vi "GamePlayfield_DetectCollision.vi"(1 "Origin":i16, 4 "Tetromino":u8, 8 "AdditionalChecks":cluster{"LeftBorder":bool, "RightBorder":bool}, 9 "Player":u8) -> (16 "Collision":bool)   [LabVIEW 2018]
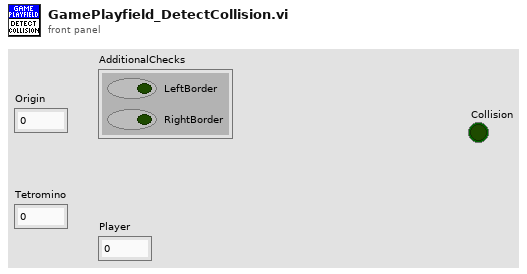
[diagram p1: front panel]
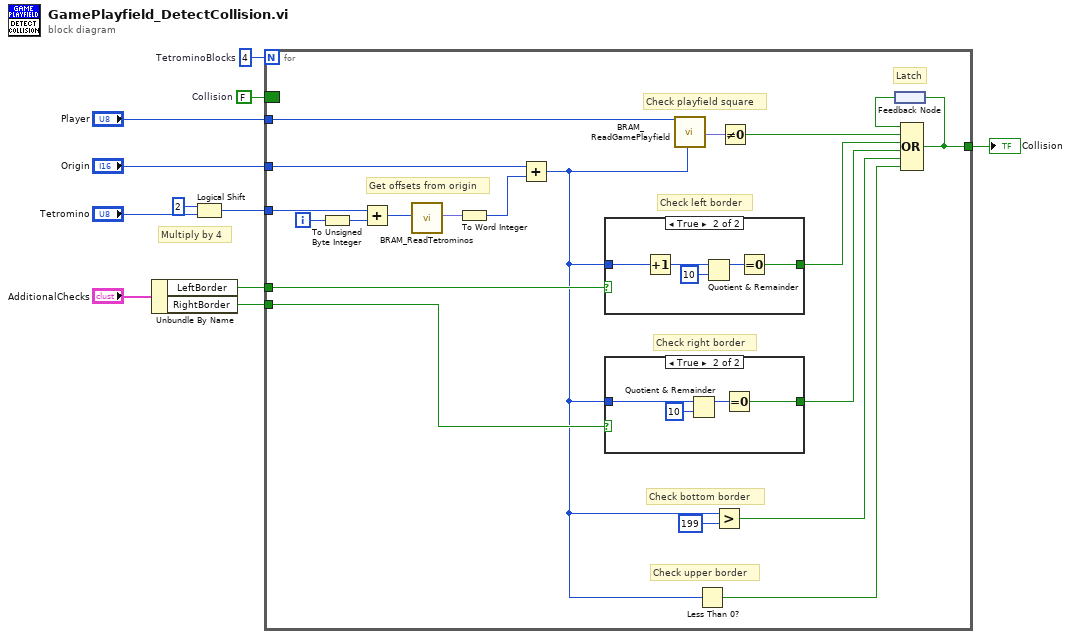
[diagram p0: block diagram]
diagram:
  w5 = FALSE  # Collision
  w9 = 4  # TetrominoBlocks
  # "Multiply by 4"
  n1 = Unbundle By Name("AdditionalChecks") -> ("LeftBorder"=w2:bool, "RightBorder"=w1:bool)
  n2 = Logical Shift(y=i16 2, x="Tetromino") -> (x << y=w8:u8)
  n3 = for {
    N: w9 -> [_]
    tunnel: w8 -> [w30]
    tunnel: "Origin" -> [w27]
    tunnel: [w24] -> w6
    border: w5 -> [_]
    tunnel: "Player" -> [w31]
    tunnel: w2 -> [w17]
    tunnel: w1 -> [w16]
    i -> [w29]
    # "Check upper border"
    # "Get offsets from origin"
    # "Check bottom border"
    # "Check right border"
    # "Check left border"
    # "Check playfield square"
    # "Latch"
    n4 = To Unsigned Byte Integer(number=w29) -> (unsigned 8bit integer=w28:u8)
    n5 = Add(x=w30, y=w28) -> (x+y=w21:u8)
    n6 = call "BRAM_ReadTetrominos.vi"("Address"=w21) -> ("Data"=w26:fxp<+,6,6>)  [unwired: 18 in]
    n7 = To Word Integer(number=w26) -> (16bit integer=w22:i16)
    n8 = Add(x=w27, y=w22) -> (x+y=w13:i16)
    n9 = case shown="True" w17 {
      tunnel: [_ w38] -> w23
      tunnel: w13 -> [_ w36]
      frame False {
      }
      frame True {
        n10 = Increment(x=w36) -> (x+1=w37:i16)
        n11 = Quotient & Remainder(x=w37, y=i16 10) -> (x-y*floor(x/y)=w40:i16)  [unwired: 1 out]
        n12 = Equal To 0?(x=w40) -> (x = 0?=w38:bool)
      }
    }
    n13 = case shown="True" w16 {
      tunnel: [_ w33] -> w18
      tunnel: w13 -> [_ w32]
      frame False {
      }
      frame True {
        n14 = Quotient & Remainder(x=w32, y=i16 10) -> (x-y*floor(x/y)=w35:i16)  [unwired: 1 out]
        n15 = Equal To 0?(x=w35) -> (x = 0?=w33:bool)
      }
    }
    n16 = call "BRAM_ReadGamePlayfield.vi"("Player IN"=w31, "Address"=w13) -> ("Data"=w19:fxp<+,3,3>)  [unwired: 16 in, 1 out]
    n17 = Less Than 0?(x=w13) -> (x < 0?=w14:bool)
    n18 = Greater?(x=w13, y=i16 199) -> (0:w15:bool)
    n19 = Not Equal To 0?(x=w19) -> (x != 0?=w20:bool)
    n20 = feedback #1() -> (w25:bool)
    n21 = Compound Arithmetic op=OR(w25, w20, w23, w18, w15, w14) -> (w24:bool)
    n22 = feedback-in #1(w24) -> ()
  }
  "Collision" <- w6
